vi "manual_test_random.vi"(7 "step_references":T1, 8 "error in (no error)":errorcluster, 11 "data":variant) -> (0 "error out":errorcluster)   [LabVIEW 2015, in "lv-recipe-machine.lvlib"]
uses:
  lv-recipe-machine.lvlib
  public/_controls/step_references.ctl
  lv-recipe-machine_/public/_controls/references.ctl
  lv-recipe-machine_/private/_controls/input.ctl
  lv-recipe-machine_/private/_controls/input_command.ctl
  lv-recipe-machine_/private/_controls/output.ctl
  lv-recipe-machine_/private/_controls/data.ctl
  lv-recipe-machine_/public/_controls/configuration.ctl
  private/_controls/recipe_data.ctl
  public/_controls/mode.ctl
  public/_controls/manual_state.ctl
  public/_controls/automatic_state.ctl
  <userlib>/antonio-alexander/lv-waitgroup/public/_controls/api_waitgroup.ctl
  public/_controls/transition.ctl
  lv-recipe-machine_/public/_controls/change.ctl
  lv-recipe-machine_/public/_controls/status.ctl
  lv-recipe-machine_/repub-dvr_nre.lvlib
  <userlib>/antonio-alexander/lv-waitgroup/lv-waitgroup.lvlib
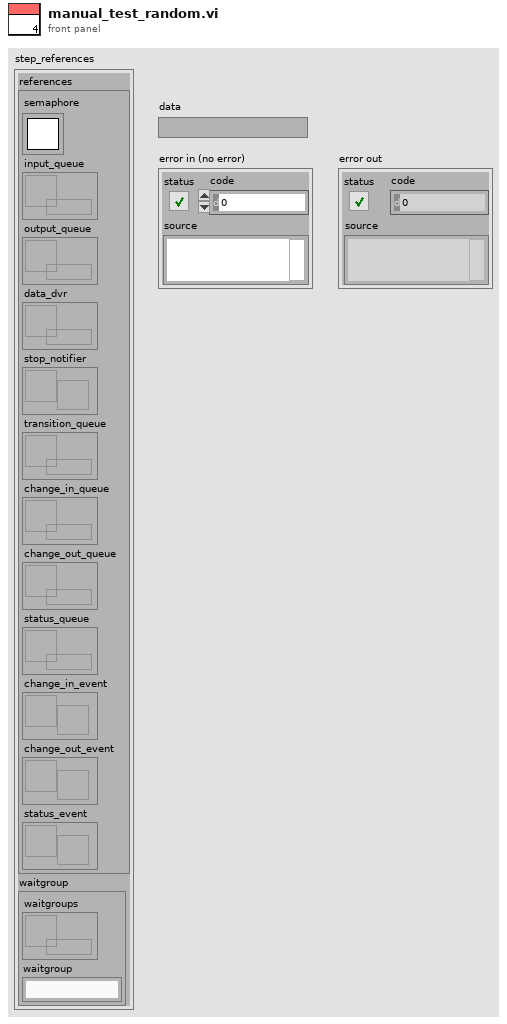
[diagram p1: front panel]
types:
  T1 = typedef "lv-recipe-machine.lvlib/step_references.ctl" = cluster{"references":T2, "api_waitgroup":T4}
  T2 = typedef "repub-dvr_nre.lvlib/references.ctl" = cluster{"semaphore":T3, "input_queue":refnum<queue>, "output_queue":refnum<queue>, "data_dvr":refnum<data-value>, "stop_notifier":refnum<notifier>, "transition_queue":refnum<queue>, "change_in_queue":refnum<queue>, "change_out_queue":refnum<queue>, "status_queue":refnum<queue>, "change_in_event":refnum<user-event>, "change_out_event":refnum<user-event>, "status_event":refnum<user-event>}
  T3 = typedef "Semaphore RefNum" = refnum<k1>
  T4 = typedef "lv-waitgroup.lvlib/api_waitgroup.ctl" = cluster{"waitgroups":refnum<data-value>, "waitgroup":string}
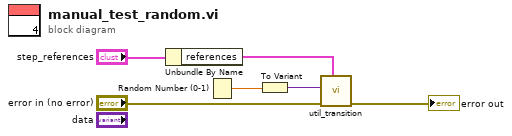
[diagram p0: block diagram]
diagram:
  n1 = Unbundle By Name("step_references") -> ("references"=w6:T2)
  n2 = Random Number (0-1)() -> (number: 0 to 1=w2:dbl)
  n3 = To Variant(anything=w2) -> (Variant=w1:variant)
  n4 = call "util_transition.vi"("references"=w6, "error in (no error)"="error in (no error)", "data"=w1) -> ("error out"=→"error out":errorcluster)  [unwired: 8 in]
